vi "SCA_init.vi"(0 "runtime(秒)":u16=10, 1 "单道1道宽":u16=3000, 2 "单道1阈值电压":u16=100) -> ()   [LabVIEW 2014]
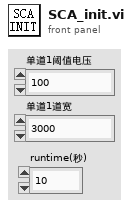
[diagram p1: front panel]
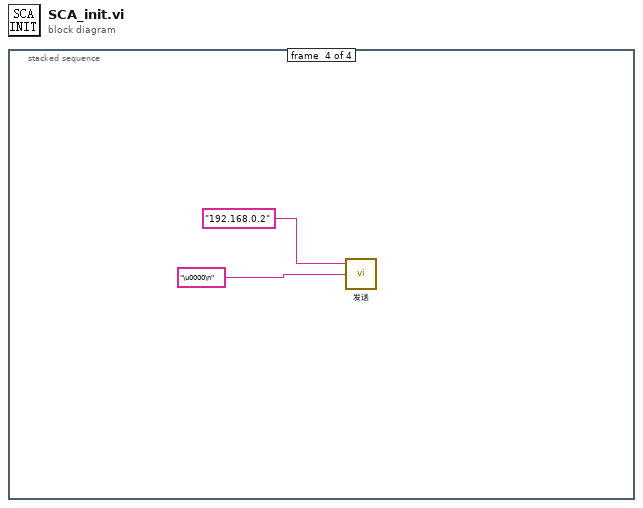
[diagram p0: block diagram]
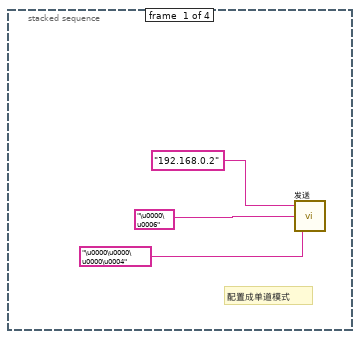
[diagram p2: hidden frame]
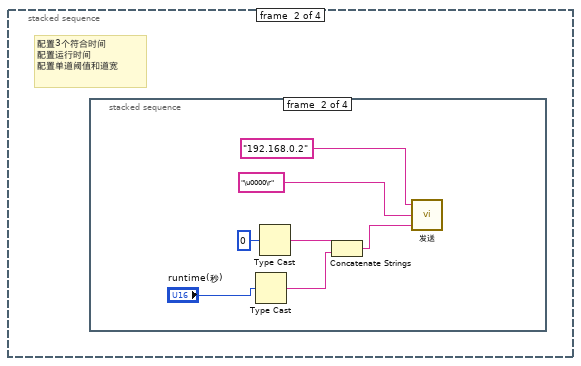
[diagram p3: hidden frame]
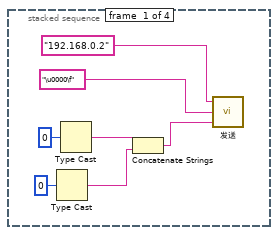
[diagram p4: hidden frame]
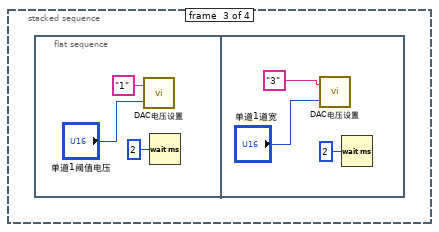
[diagram p5: hidden frame]
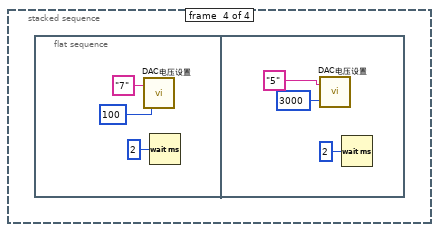
[diagram p6: hidden frame]
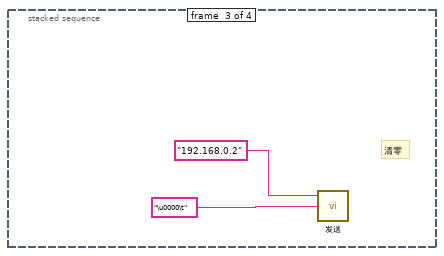
[diagram p7: hidden frame]
diagram:
  n1 = stacked-sequence {
    frame #0 {
      # "配置成单道模式"
      n2 = call "发送.vi"("数据（32bit）"="\u0000\u0000\u0000\u0004", "命令(16bit)"="\u0000\u0006", "目标IP"="192.168.0.2") -> ()  [unwired: 1 out]
    }
    frame #1 {
      # "配置3个符合时间\n配置运行时间\n配置单道阈值和道宽"
      n3 = stacked-sequence {
        frame #0 {
          n4 = Type Cast(x=u16 0) -> (*(type *) &x=w6:string)  [unwired: 1 in]
          n5 = Type Cast(x=u16 0) -> (*(type *) &x=w7:string)  [unwired: 1 in]
          n6 = Concatenate Strings(w7, w6) -> (w8:string)
          n7 = call "发送.vi"("数据（32bit）"=w8, "命令(16bit)"="\u0000\f", "目标IP"="192.168.0.2") -> ()  [unwired: 1 out]
        }
        frame #1 {
          n8 = Type Cast(x="runtime(秒)") -> (*(type *) &x=w13:string)  [unwired: 1 in]
          n9 = Type Cast(x=u16 0) -> (*(type *) &x=w14:string)  [unwired: 1 in]
          n10 = Concatenate Strings(w14, w13) -> (w15:string)
          n11 = call "发送.vi"("数据（32bit）"=w15, "命令(16bit)"="\u0000\r", "目标IP"="192.168.0.2") -> ()  [unwired: 1 out]
        }
        frame #2 {
          n12 = flat-sequence {
            frame #0 {
              n13 = call "DAC电压设置.vi"("电压"="单道1阈值电压", "cmd_channel(8bit)"="1") -> ()  [unwired: 1 in]
              n14 = Wait (ms)(milliseconds to wait=u32 2 ("等待时间（毫秒）")) -> ()  [unwired: 1 out]
            }
            frame #1 {
              n15 = call "DAC电压设置.vi"("电压"="单道1道宽", "cmd_channel(8bit)"="3") -> ()  [unwired: 1 in]
              n16 = Wait (ms)(milliseconds to wait=u32 2 ("等待时间（毫秒）")) -> ()  [unwired: 1 out]
            }
          }
        }
        frame #3 {
          n17 = flat-sequence {
            frame #0 {
              n18 = call "DAC电压设置.vi"("电压"=u16 100, "cmd_channel(8bit)"="7") -> ()  [unwired: 1 in]
              n19 = Wait (ms)(milliseconds to wait=u32 2 ("等待时间（毫秒）")) -> ()  [unwired: 1 out]
            }
            frame #1 {
              n20 = call "DAC电压设置.vi"("电压"=u16 3000, "cmd_channel(8bit)"="5") -> ()  [unwired: 1 in]
              n21 = Wait (ms)(milliseconds to wait=u32 2 ("等待时间（毫秒）")) -> ()  [unwired: 1 out]
            }
          }
        }
      }
    }
    frame #2 {
      # "清零"
      n22 = call "发送.vi"("命令(16bit)"="\u0000\t", "目标IP"="192.168.0.2") -> ()  [unwired: 1 in, 1 out]
    }
    frame #3 {
      n23 = call "发送.vi"("命令(16bit)"="\u0000\n", "目标IP"="192.168.0.2") -> ()  [unwired: 1 in, 1 out]
    }
  }
